vi "Shutter and DMD OG.vi"(4 "PFI 0 digital clock frequency":dbl, 5 "sCMOS fps":dbl, 6 "OG repitation":dbl, 7 "Objective 线性减速 时间（s）":dbl, 8 "Objective volet 线性减速 时间（s）":dbl, 9 "Objective 刺激steps 时间（s）":dbl, 10 "Objective 线性加速 时间（s）":dbl) -> (2 "DMD OG digital output":bool[](array[boolean]), 3 "Shutter OG digital output":bool[](array[boolean]))   [LabVIEW 2018]
panel:
  out "New":i32
  out "new":dbl
  out "old":i32
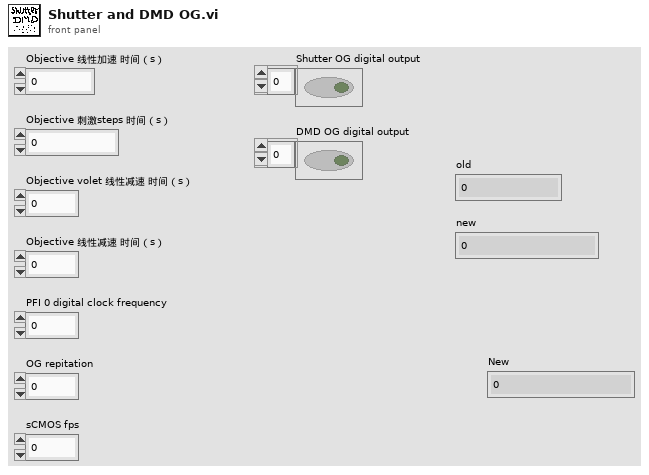
[diagram p1: front panel]
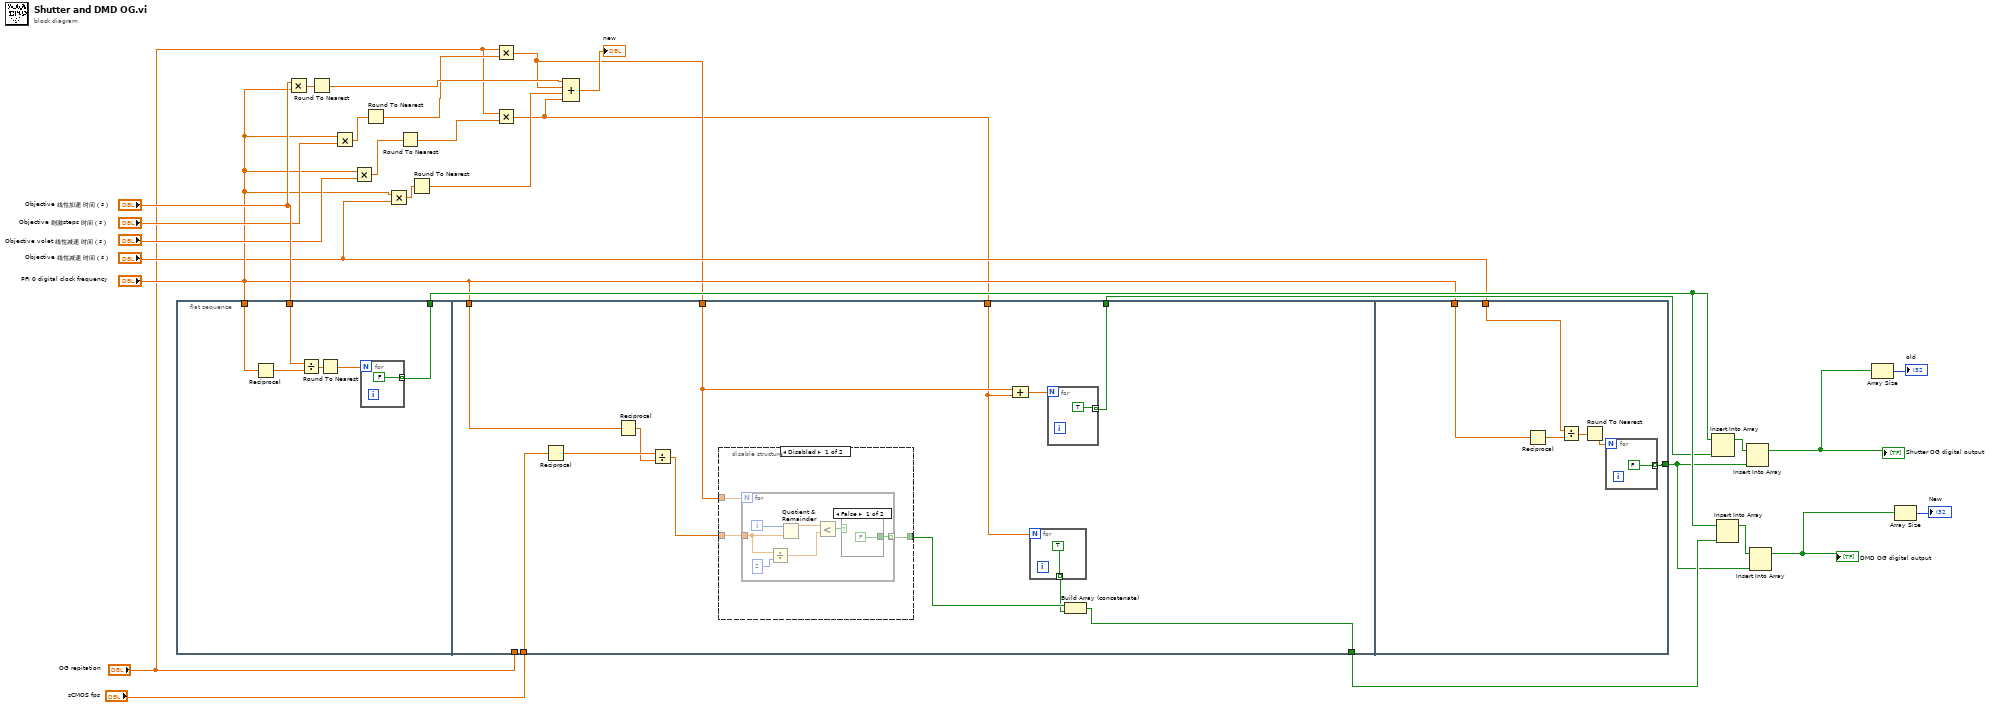
[diagram p0: block diagram]
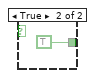
[diagram p2: hidden frame]
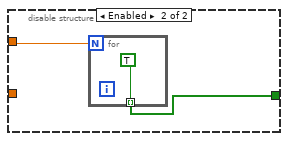
[diagram p3: hidden frame]
diagram:
  n1 = flat-sequence {
    tunnel: [w31] -> w25
    tunnel: "Objective 线性加速 时间（s）" -> [w30]
    tunnel: "PFI 0 digital clock frequency" -> [w29]
    tunnel: [w47] -> w22
    tunnel: [w39] -> w27
    tunnel: "PFI 0 digital clock frequency" -> [w43]
    tunnel: "OG repitation" -> [_]
    tunnel: "sCMOS fps" -> [w42]
    tunnel: w4 -> [w38]
    tunnel: w3 -> [w37]
    tunnel: [w67] -> w24
    tunnel: "Objective 线性减速 时间（s）" -> [w66]
    tunnel: "PFI 0 digital clock frequency" -> [w65]
    frame #0 {
      n2 = Reciprocal(x=w29) -> (1/x=w34:dbl)
      n3 = Divide(x=w30, y=w34) -> (x/y=w33:dbl)
      n4 = Round To Nearest(number=w33) -> (nearest integer value=w32:dbl)
      n5 = for {
        N: w32 -> [_]
        tunnel: [FALSE] -> w31 mode=indexing
      }
    }
    frame #1 {
      n6 = Reciprocal(x=w42) -> (1/x=w46:dbl)
      n7 = Reciprocal(x=w43) -> (1/x=w44:dbl)
      n8 = Divide(x=w46, y=w44) -> (x/y=w45:dbl)
      n9 = disable-structure shown="Disabled" {
        disable-tunnel: w45 -> [w50 _]
        disable-tunnel: w38 -> [w49 w61]
        disable-tunnel: [w48 w60] -> w41
        frame Disabled {
          n10 = for {
            N: w49 -> [_]
            tunnel: w50 -> [w56]
            tunnel: [w51] -> w48 mode=indexing
            i -> [w57]
            n11 = Divide(x=w56, y=2) -> (x/y=w53:dbl)
            n12 = Quotient & Remainder(x=w57, y=w56) -> (x-y*floor(x/y)=w54:dbl)  [unwired: 1 out]
            n13 = Less?(x=w54, y=w53) -> (x < y?=w52:bool)
            n14 = case shown="False" w52 {
              tunnel: [FALSE TRUE] -> w51
              frame False {
              }
              frame True {
              }
            }
          }
        }
        frame Enabled {
          n15 = for {
            N: w61 -> [_]
            tunnel: [TRUE] -> w60 mode=indexing
          }
        }
      }
      n16 = Compound Arithmetic op=ADD(w38, w37) -> (w36:dbl)
      n17 = for {
        N: w37 -> [_]
        tunnel: [TRUE] -> w40 mode=indexing
      }
      n18 = for {
        N: w36 -> [_]
        tunnel: [TRUE] -> w47 mode=indexing
      }
      n19 = Build Array (concatenate)(w41, w40) -> (w39:bool[])
    }
    frame #2 {
      n20 = Reciprocal(x=w65) -> (1/x=w70:dbl)
      n21 = Divide(x=w66, y=w70) -> (x/y=w69:dbl)
      n22 = Round To Nearest(number=w69) -> (nearest integer value=w68:dbl)
      n23 = for {
        N: w68 -> [_]
        tunnel: [FALSE] -> w67 mode=indexing
      }
    }
  }
  n24 = Multiply(x="Objective 线性加速 时间（s）", y="PFI 0 digital clock frequency") -> (x*y=w14:dbl)
  n25 = Round To Nearest(number=w14) -> (nearest integer value=w10:dbl)
  n26 = Multiply(x="PFI 0 digital clock frequency", y="Objective 刺激steps 时间（s）") -> (x*y=w13:dbl)
  n27 = Multiply(x="PFI 0 digital clock frequency", y="Objective volet 线性减速 时间（s）") -> (x*y=w12:dbl)
  n28 = Round To Nearest(number=w13) -> (nearest integer value=w7:dbl)
  n29 = Multiply(x="PFI 0 digital clock frequency", y="Objective 线性减速 时间（s）") -> (x*y=w11:dbl)
  n30 = Round To Nearest(number=w12) -> (nearest integer value=w5:dbl)
  n31 = Round To Nearest(number=w11) -> (nearest integer value=w9:dbl)
  n32 = Multiply(x="OG repitation", y=w7) -> (x*y=w4:dbl)
  n33 = Multiply(x="OG repitation", y=w5) -> (x*y=w3:dbl)
  n34 = Compound Arithmetic op=ADD(w10, w4, w9, w3) -> (→"new":dbl)
  n35 = Insert Into Array(array=w25, new element=w22) -> (w23:bool[])  [unwired: 1 in]
  n36 = Insert Into Array(array=w25, new element=w27) -> (w26:bool[])  [unwired: 1 in]
  n37 = Insert Into Array(array=w23, new element=w24) -> (w21:bool[])  [unwired: 1 in]
  "Shutter OG digital output" <- w21
  n38 = Insert Into Array(array=w26, new element=w24) -> (w1:bool[])  [unwired: 1 in]
  "DMD OG digital output" <- w1
  n39 = Array Size(array=w21) -> (size(s)=→"old":i32)
  n40 = Array Size(array=w1) -> (size(s)=→"New":i32)
